vi "CheckDeviceID.vi"(8 "error in (no error)":errorcluster, 11 "ColorSensorDevRef":T1={"I2CDevRef"={"DevStatus"={"status"=FALSE, "code"=0, "source"=""}, "Device Address"=0, "Handle"=0, "I2C Bus"=enum."Invalid"}} {"I2CDevRef"."Device Address" format="%.0x"}) -> (0 "error out":errorcluster, 2 "Correct?":bool, 3 "ColorSensorDevRef out":T1={"I2CDevRef"={"DevStatus"={"status"=FALSE, "code"=0, "source"=""}, "Device Address"=0, "Handle"=0, "I2C Bus"=enum."Invalid"}} {"I2CDevRef"."Device Address" format="%.0x"})   [LabVIEW 2018, in "ColorSensor.lvlib"]
uses:
  ColorSensor.lvlib
  ColorSensorDevRef.ctl
  <vilib>/Rock Robotics/WPI/I2C/WPI_I2CDevRef.ctl
  <vilib>/Rock Robotics/SystemInterfaces/i2clib/i2c_bus.ctl
panel:
  out "PartID":u8[](array[numeric])
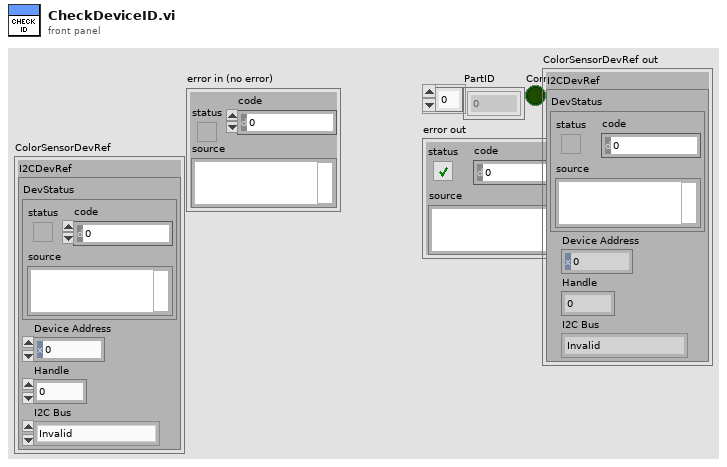
[diagram p1: front panel]
types:
  T1 = typedef "ColorSensor.lvlib/ColorSensorDevRef.ctl" = cluster{"I2CDevRef":T2}
  T2 = typedef "WPI_I2CDevRef.ctl" = cluster{"DevStatus":errorcluster, "Device Address":u8, "Handle":i32, "I2C Bus":T3}
  T3 = typedef "i2c_bus.ctl" = enum16{"I2C On-Board", "I2C MXP", "Invalid"}
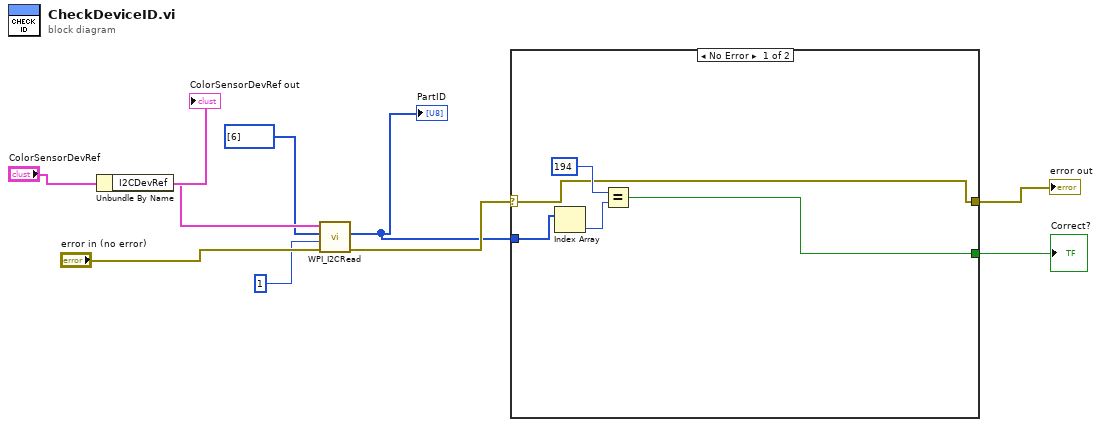
[diagram p0: block diagram]
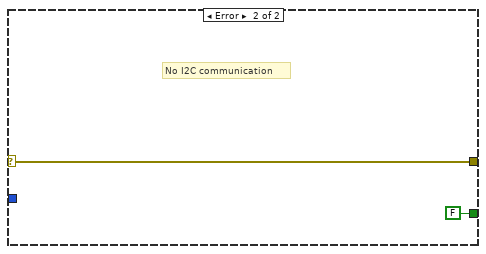
[diagram p2: hidden frame]
diagram:
  n1 = Unbundle By Name("ColorSensorDevRef") -> ("I2CDevRef"=w8:T2)
  n2 = call <vilib>:"WPI_I2CRead.vi"("error in (no error)"="error in (no error)", "I2CBytesToRead"=u8 1, "I2CRegister"=u8[] [6], "I2CDevRef"=w8) -> ("error out"=w4:errorcluster, "Data Out"=w3:u8[])  [unwired: 5 in, 1 out]
  "PartID" <- w3
  n3 = case shown="No Error" w4 {
    selector: w4 -> [w10 w16]
    tunnel: w3 -> [w14 _]
    tunnel: [w10 w16] -> w2
    tunnel: [w11 FALSE] -> w1
    frame No Error {
      n4 = Index Array(array=w14) -> (element=w13:u8)  [unwired: 1 in]
      n5 = Equal?(x=u8 194, y=w13) -> (x = y?=w11:bool)
    }
    frame Error {
      # "No I2C communication"
    }
  }
  "error out" <- w2
  "Correct?" <- w1
  "ColorSensorDevRef out" <- "ColorSensorDevRef"
